vi "Select HDF5 Dialog (File and Object).vi"(0 "Initial File Path":path, 2 "Item Filters":T5 {"Object Types (any)" items=["H5G_UNKNOWN"=-1, "H5G_GROUP"=0, "H5G_DATASET"=1, "H5G_TYPE"=2, "H5G_LINK"=3, "H5G_UDLINK"=4]}, 3 "File Browse Options":T8, 5 "Close HDF5 File?":bool, 7 "Initial Object Path":string, 11 "error in":errorcluster, 12 "Operation Modes":cluster{"File":T2, "Object":T3}={"File"=enum."open or create", "Object"=enum."open or create"}, 13 "Window":T7={"Behavior"=enum."Modal", "Position"={"Left"=0, "Top"=0, "Right"=600, "Bottom"=400}, "Center"=TRUE, "Title"="Select an HDF5 Object"}) -> (4 "File Path out":path, 6 "HDF5 File Ref out":T1, 8 "Object Path out":string, 10 "OK?":bool, 14 "Object operation out":T9(ring), 15 "error out":errorcluster)   [LabVIEW 2017]
doc: "Displays a dialog prompting the user to select a dataset, datatype,\n or group from an HDF5 file."
uses:
  <vilib>/Utility/miscctls.llb/LVRectTypeDef.ctl
  <vilib>/UPVI/lvhdf5/group.llb/H5G_obj_t.ctl
  <vilib>/UPVI/lvhdf5/file.llb/LVH5F Operation.ctl
  <vilib>/UPVI/lvhdf5/dataset.llb/LVH5D Operation.ctl
  <vilib>/UPVI/lvhdf5/library.llb/HDF5 Ref.ctl
panel:
  # "LVHDF5 Toolkit\nCopyright (c) 2005-2013 by Jason D. Sommerville\nCopyright (c) 2014 by UPVI, LLC.\n\nThis use and distribution of this file is governed by the terms found in \nLICENSE.txt distributed with this toolkit and installed at\n <user.lib>\\_lvhdf5\\LICENSE.txt"
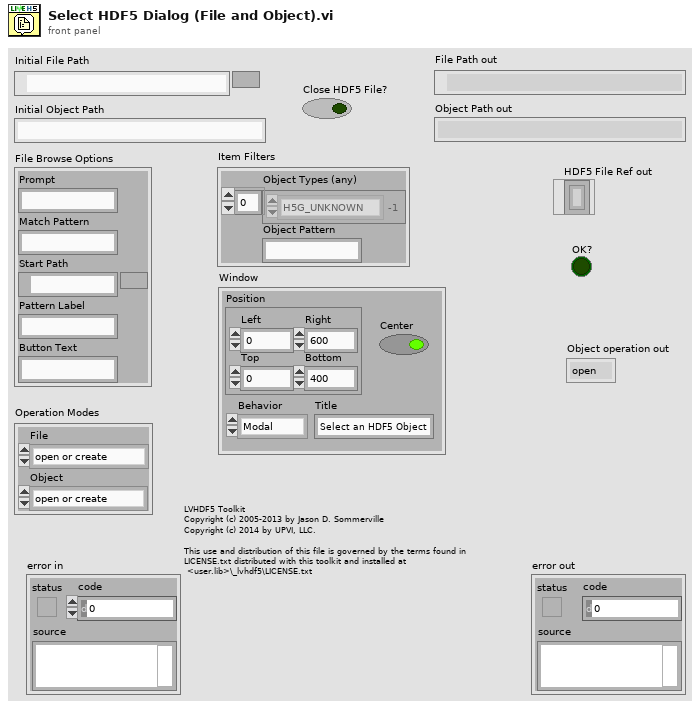
[diagram p1: front panel]
types:
  T1 = typedef "HDF5 Ref.ctl" = refnum<k1>
  T2 = typedef "LVH5F Operation.ctl" = enum16{"open", "open or create", "create or replace", "create or replace (with confirmation)", "create", "open (read only)"}
  T3 = typedef "LVH5D Operation.ctl" = enum16{"open", "replace", "create", "open or create", "create or replace", "create or replace with confirmation"}
  T4 = typedef "H5G_obj_t.ctl" = i32
  T5 = cluster{"Object Types (any)":T4[], "Object Pattern":string}
  T6 = typedef "LVRectTypeDef.ctl" = cluster{"Left":i16, "Top":i16, "Right":i16, "Bottom":i16}
  T7 = cluster{"Behavior":enum32{"Invalid", "Default", "Floating", "Floating/Auto-Hide", "Modal"}, "Position":T6, "Center":bool, "Title":string}
  T8 = cluster{"Prompt":string, "Match Pattern":string, "Start Path":path, "Pattern Label":string, "Button Text":string}
  T9 = enum16{"open", "replace", "create", "open or create", "replace or create", "replace or create with confirmation"}
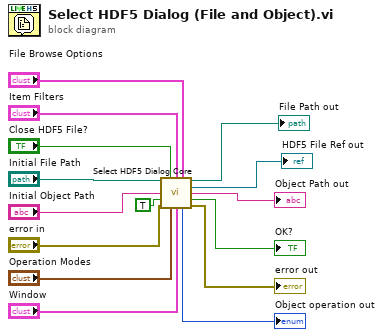
[diagram p0: block diagram]
diagram:
  n1 = call <vilib>:"Select HDF5 Dialog Core.vi"("Initial File Path"="Initial File Path", "Close HDF5 File?"="Close HDF5 File?", "Item Filters"="Item Filters", "File Browse Options"="File Browse Options", "Initial Object Path"="Initial Object Path", "Path visible"=TRUE, "error in"="error in", "Operation Modes"="Operation Modes", "Window"="Window") -> ("File Path out"=→"File Path out":path, "HDF5 File Ref out"=→"HDF5 File Ref out":T1, "Object Path out"=→"Object Path out":string, "OK?"=→"OK?":bool, "Object operation out"=→"Object operation out":T9, "error out"=→"error out":errorcluster)  [unwired: 1 in]
